vi "RW_VoltageTest.vi"(0 "datain":string[](array[string])=["备注", "负载通道", "负载地址", "延时时间", "output max", "output min", "量测类型", "待测物板号"], 5 "HW CH Number":i32, 7 "Setup":string) -> (4 "REPORT INDECATE":string[][](array[string])=[["微安测试", "", "", "", ""], ["微安量测", "4", "0.000", "0.1", "NG"], ["微安量测", "4", "0.000", "0.1", "NG"], ["微安量测", "4", "0.000", "0.1", "NG"], ["微安量测", "4", "0.000", "0.1", "NG"]], 6 "ROW HEAD":string[](array[string]), 8 "PF":string[](array[string]), 10 "testData":string[](array[string]), 15 "Array":string[](array[string]))   [LabVIEW 2018]
panel:
  out "测试板数":i32
  out "数组":bool[](array[boolean])
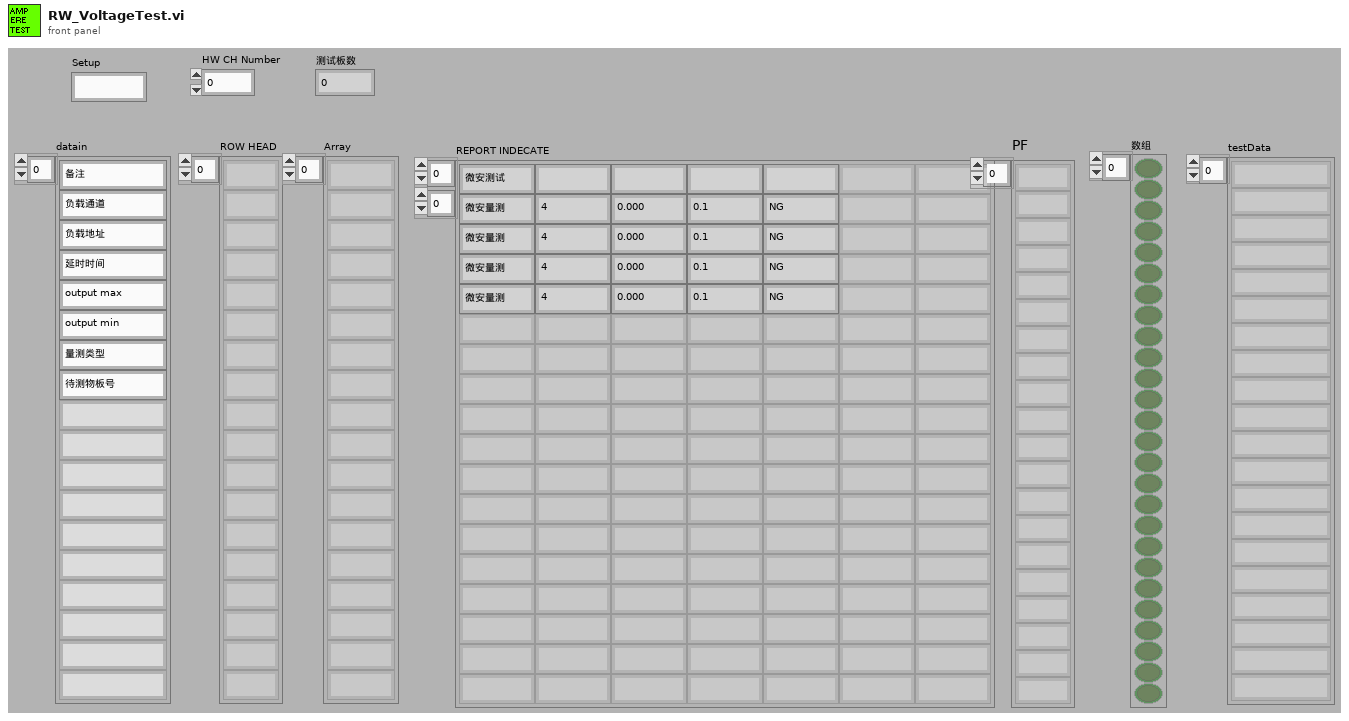
[diagram p1: front panel]
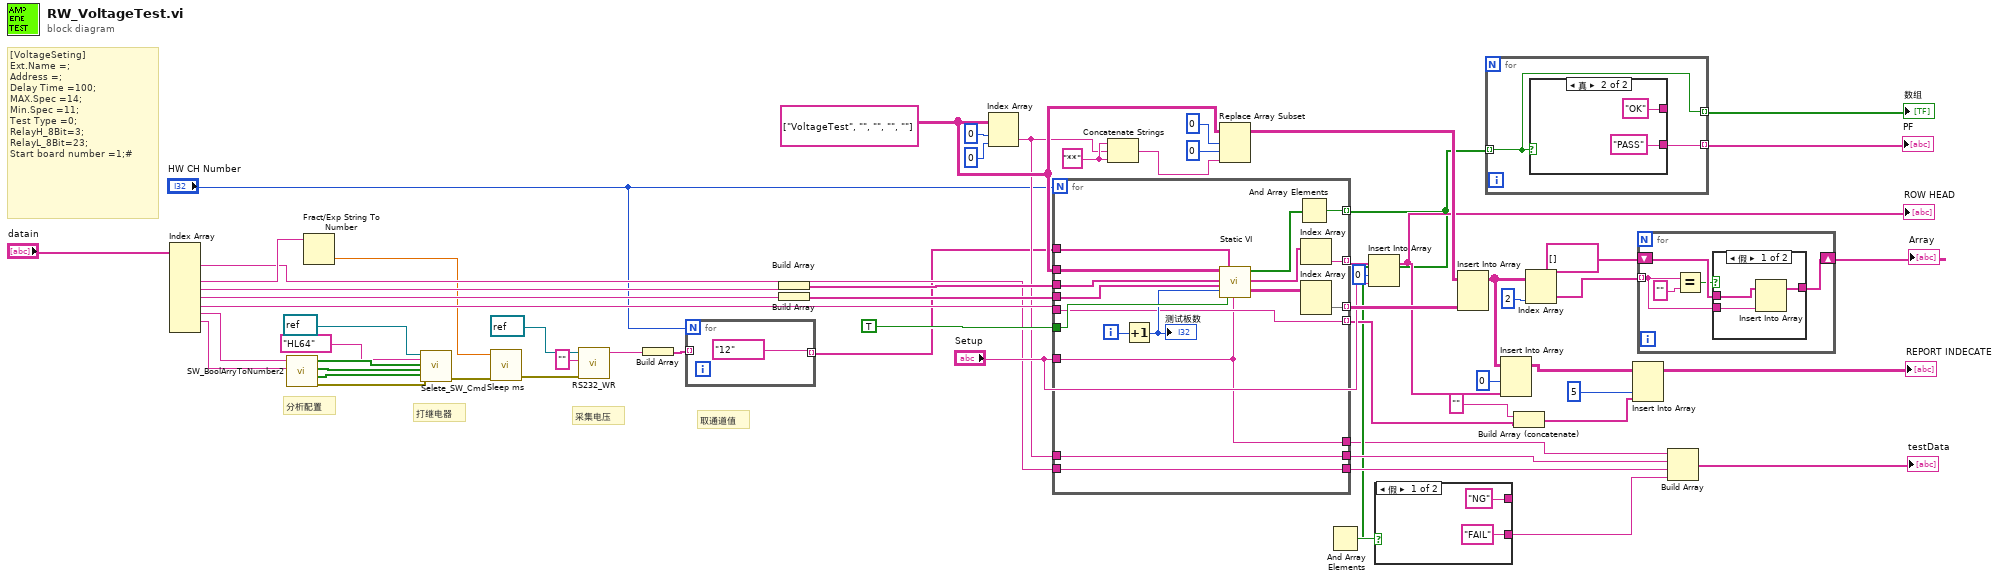
[diagram p0: block diagram]
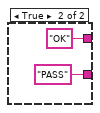
[diagram p2: hidden frame]
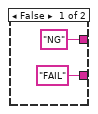
[diagram p3: hidden frame]
diagram:
  w46 = string[][] [["VoltageTest", "", "", "", ""]]
  w52 = "**" ("字符串")
  # "取通道值"
  # "分析配置"
  # "打继电器"
  # "采集电压"
  # "[VoltageSeting]\nExt.Name =;\nAddress =;\nDelay Time =100;\nMAX.Spec =14;\nMin.Spec =11;\nTest Type =0;\nRelayH_8Bit=3;\nRelayL_8Bit=23;\nStart board number =1;#"
  n1 = Index Array(array="datain") -> (element #1=w26:string, element #3=w55:string, element #4=w48:string, element #5=w47:string, element #6=w34:string, element #7=w16:string, element #8=w17:string)  [unwired: 9 in, 2 out]
  n2 = call "SW_BoolArryToNumber2.vi"("L32 INUPT"=w17, "H32 INUPT"=w16) -> ("error out"=w15:errorcluster, "64 SW OUT"=w14:bool[], "L_32"=w13:bool[], "H_32"=w12:bool[])  [unwired: 6 in]
  n3 = Fract/Exp String To Number(string=w55) -> (number=w1:dbl)  [unwired: 3 in, 1 out]
  n4 = call "Selete_SW_Cmd.vi"("VISA资源名称 2"=refnum<visa-resource-name> refnum ("VISA资源名称"), "组合框"="HL64", "H_32"=w12, "L_32"=w13, "64 SW OUT"=w14, "error in (no error)"=w15) -> ("error out"=w9:errorcluster)  [unwired: 12 in, 1 out]
  n5 = call "Sleep ms.vi"("error in (no error)"=w9, "等待时间（毫秒）"=w1) -> ("error out"=w6:errorcluster)  [unwired: 9 in]
  n6 = call "RS232_WR.vi"("error in (no error)"=w6, "CMD"="", "VISA资源名称"=refnum<visa-resource-name> refnum) -> ("读取缓冲区"=w5:string)  [unwired: 6 in, 2 out]
  n7 = Build Array(w5) -> (w4:string[])
  n8 = for {
    N: "HW CH Number" -> [_]
    tunnel: w4 -> [_] mode=indexing
    tunnel: ["12" ("F-格式字符串")] -> w2 mode=indexing
  }
  n9 = Build Array(w48) -> (w45:string[])
  n10 = Build Array(w47) -> (w44:string[])
  n11 = Index Array(array=w46, index (row)=0 ("索引 (行)"), index (col)=0 ("禁用的索引 (列)")) -> (element=w27:string)
  n12 = for {
    N: "HW CH Number" -> [_]
    tunnel: w2 -> [w79]
    tunnel: w45 -> [w77]
    tunnel: w44 -> [w76]
    tunnel: "Setup" -> [w63]
    tunnel: TRUE -> [w74]
    tunnel: [w72] -> w22 mode=indexing
    tunnel: [w69] -> w40 mode=indexing
    tunnel: w46 -> [w78]
    tunnel: [w67] -> w41 mode=indexing
    tunnel: w34 -> [w66]
    tunnel: [w66] -> w30 mode=indexing
    tunnel: w27 -> [w65]
    tunnel: [w65] -> w25
    tunnel: w26 -> [w64]
    tunnel: [w64] -> w24
    tunnel: [w63] -> w19
    i -> [w71]
    n13 = Increment(x=w71) -> (x+1=w73:i32)
    "测试板数" <- w73
    n14 = call "Static VI.vi"("添加的数组"=w78, "Max"=w77, "Min"=w76, "板数"=w73, "INPUTSTRING"=w79, "是否为字符串对比"=w74, "SQ"=w63) -> ("P/F"=w75:bool[], "SQ out"=w70:string[], "arrauy out"=w68:string[][])  [unwired: 9 in, 1 out]
    n15 = And Array Elements(Boolean array=w75) -> (logical AND=w72:bool)
    n16 = Index Array(array=w70) -> (element=w69:string)  [unwired: 1 in]
    n17 = Index Array(array=w68) -> (element=w67:string[])  [unwired: 2 in]
  }
  n18 = Concatenate Strings(w52, w27, w52) -> (w49:string)
  n19 = Replace Array Subset(array=w46, new element=w49, index (row)=0 ("索引 (行)"), index (col)=0 ("禁用的索引 (列)")) -> (w42:string[][])
  n20 = And Array Elements(Boolean array=w22) -> (logical AND=w23:bool)
  n21 = Insert Into Array(array=w40, index=0 ("索引"), new element="Setup") -> (w36:string[])
  "ROW HEAD" <- w36
  n22 = case shown="假" w23 {
    tunnel: ["NG" "OK"] -> _
    tunnel: ["FAIL" "PASS"] -> w21
    frame False {
    }
    frame True {
    }
  }
  n23 = Insert Into Array ("数组插入")(array=w42, new element=w41) -> (w37:string[][])  [unwired: 2 in]
  n24 = for {
    tunnel: w22 -> [w84] mode=indexing
    tunnel: [w85] -> w57 mode=indexing
    tunnel: [w84] -> w18 mode=indexing
    n25 = case shown="真" w84 {
      tunnel: ["NG" "OK"] -> _
      tunnel: ["FAIL" "PASS"] -> w85
      frame False {
      }
      frame True {
      }
    }
  }
  "PF" <- w57
  "数组" <- w18
  n26 = Insert Into Array(array=w37, index (col)=0 ("禁用的索引 (列)"), new element=w36) -> (w32:string[][])  [unwired: 1 in]
  n27 = Build Array (concatenate)("" ("字符串"), w30) -> (w28:string[])
  n28 = Index Array(array=w37, index (col)=2 ("禁用的索引 (列)")) -> (element=w59:string[])  [unwired: 1 in]
  n29 = Insert Into Array(array=w32, index (col)=5 ("禁用的索引 (列)"), new element=w28) -> (→"REPORT INDECATE":string[][])  [unwired: 1 in]
  n30 = for {
    tunnel: w59 -> [w90] mode=indexing
    shift-right: [w91] -> w58
    shift-left: string[] [] ("Array") -> [w94]
    n31 = Equal?(x=w90, y="") -> (x = y?=w92:bool)
    n32 = case shown="假" w92 {
      tunnel: w94 -> [w97 w98]
      tunnel: [w96 w98] -> w91
      tunnel: w90 -> [w95 _]
      frame False {
        n33 = Insert Into Array(array=w97, new element=w95) -> (w96:string[])  [unwired: 1 in]
      }
      frame True {
      }
    }
  }
  "Array" <- w58
  n34 = Build Array(w19, w25, w24, w21) -> (→"testData":string[])
